vi "setUp.vi"(8 "error in (no error)":errorcluster, 11 "reference in":refnum<class "Engine Simulation IO System Tests.lvclass">) -> (0 "error out":errorcluster, 3 "reference out":refnum<class "Engine Simulation IO System Tests.lvclass">)   [LabVIEW 2015, in "Engine Simulation IO System Tests.lvclass"]
doc: "setUp runs prior to the test method during test execution. Use this method to initialize any object data required by your tests."
uses:
  Engine Simulation IO System Tests.lvclass
  NationalInstruments.VeriStand.SystemDefinitionAPI
  Engine Simulation IO System Tests.lvclass/Engine Simulation IO System Tests.ctl
  <userlib>/_OpenG.lib/file/file.llb/Append Path to Root if Relative - Scalar__ogtk.vi
  <vilib>/addons/_JKI Toolkits/VI Tester/TestCase.llb/TestCase.lvclass
  Scripting API/Engine Simulation Toolkit Scripting API.lvlib
  System Explorer/Engine Simulation Toolkit System Explorer.lvlib
  niveristand-custom-device-testing-tools/VeriStandTestUtilities/VeriStandTestUtilities.lvlib
panel:
  in  "System Definition File":path=path "Assets/estksysdef.nivssdf"
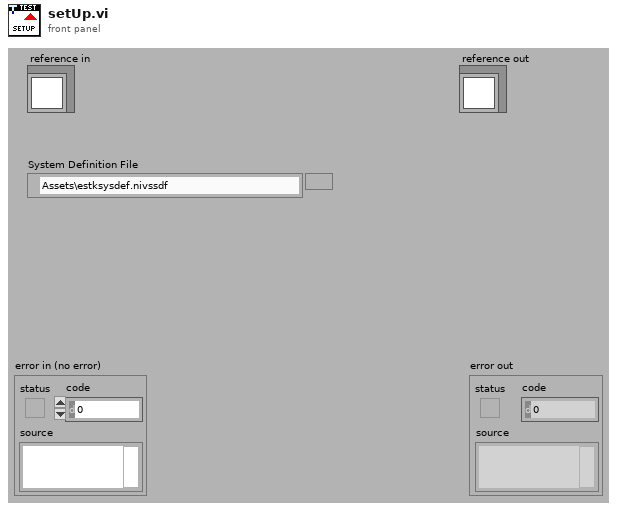
[diagram p1: front panel]
types:
  T1 = typedef "VeriStandTestUtilities.lvlib/SystemDefinitionInformation.ctl" = cluster{"Path":path, "Target Information List":T2[]}
  T2 = typedef "VeriStandTestUtilities.lvlib/TargetInformation.ctl" = cluster{"Name":string, "IP Address":string, "Operating System":string, "Target Rate":dbl, "Chassis List":T3[], "Custom Device List":string[]}
  T3 = typedef "VeriStandTestUtilities.lvlib/ChassisInformation.ctl" = cluster{"Name":string, "Devices":string[]}
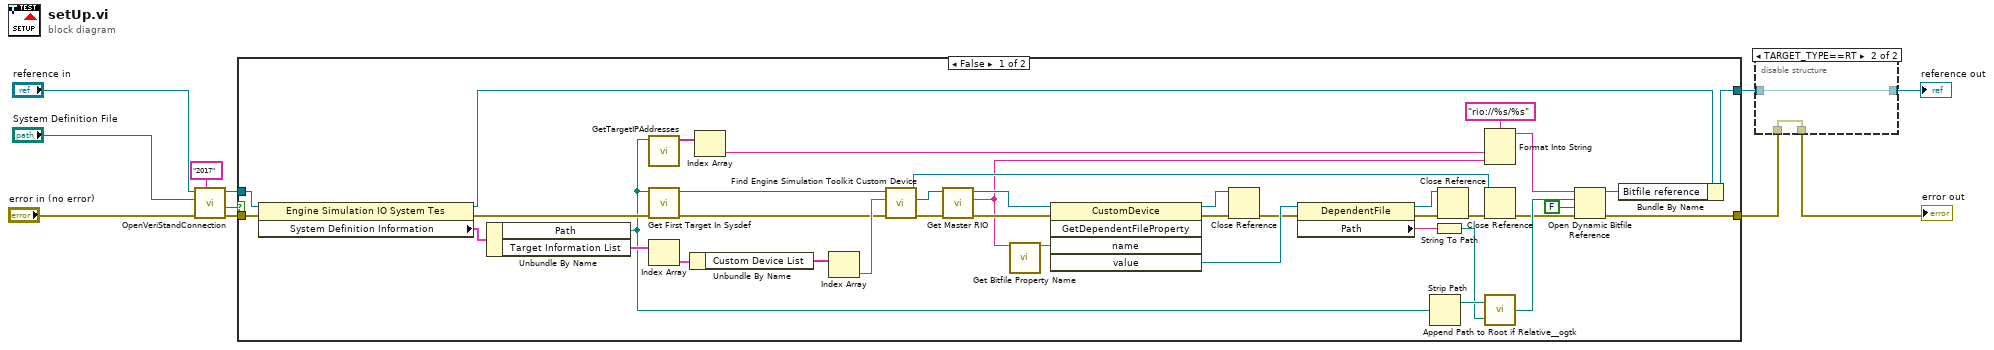
[diagram p0: block diagram]
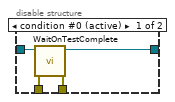
[diagram p3: hidden frame]
diagram:
  n1 = call-dynamic "OpenVeriStandConnection.vi"("Minimum VeriStand Version (2015)"="2017", "error in (no error)"="error in (no error)", "System Definition File"="System Definition File", "VeriStand Test Case in"="reference in") -> ("error out"=w5:errorcluster, "Open Skipped"=w1:bool, "VeriStand Test Case out"=w6:refnum<class "Engine Simulation IO System Tests.lvclass">)  [unwired: 5 in]
  n2 = case shown="False" w1 {
    tunnel: [w50 w51] -> w9
    tunnel: w6 -> [w49 w51]
    tunnel: w5 -> [w48 w52]
    tunnel: [w20 w52] -> w4
    frame False {
      n3 = property class="Engine Simulation IO System Tes"(reference=w49, error in=w48) -> (reference out=w12:refnum<class "Engine Simulation IO System Tests.lvclass">, error out=w46:errorcluster, "System Definition Information"=w47:T1)
      n4 = Unbundle By Name(w47) -> ("Path"=w16:path, "Target Information List"=w26:T2[])
      n5 = call "GetTargetIPAddresses.vi"("absolute system definition file"=w16) -> ("ip addresses"=w15:string[])  [unwired: 9 in, 1 out]
      n6 = call "Get First Target In Sysdef.vi"("error in (no error)"=w46, "Sysdef Path"=w16) -> ("error out"=w24:errorcluster, "Target"=w25:refnum<k24>)  [unwired: 8 in]
      n7 = Index Array(array=w26) -> (element=w45:T2)  [unwired: 1 in]
      n8 = Unbundle By Name(w45) -> ("Custom Device List"=w44:string[])
      n9 = Index Array(array=w15) -> (element=w14:string)  [unwired: 1 in]
      n10 = Index Array(array=w44) -> (element=w43:string)  [unwired: 1 in]
      n11 = call "Find Engine Simulation Toolkit Custom Device.vi"("error in (no error)"=w24, "Name"=w43, "Target in"=w25) -> ("error out"=w38:errorcluster, "EST Custom Device"=w40:refnum<k24>, "Target out"=w42:refnum<k24>)  [unwired: 6 in]
      n12 = call "Get Master RIO.vi"("error in (no error)"=w38, "EST Custom Device in"=w40) -> ("error out"=w37:errorcluster, "RIO Device Address"=w17:string, "EST Custom Device out"=w35:refnum<k24>)  [unwired: 7 in]
      n13 = call "Get Bitfile Property Name.vi"("RIO Device Address in"=w17) -> ("Bitfile Property Name"=w39:string)  [unwired: 10 in]
      n14 = invoke class="CustomDevice" method="GetDependentFileProperty"(reference=w35, error in=w37, "name"=w39) -> (reference out=w33:refnum<k24>, error out=w34:errorcluster, "value"=w41:refnum<k24>)  [unwired: 2 in, 2 out]
      n15 = Close Reference(reference=w33, error in (no error)=w34) -> (error out=w32:errorcluster)
      n16 = property class="DependentFile"(reference=w41, error in=w32) -> (reference out=w30:refnum<k24>, error out=w31:errorcluster, "Path"=w36:string)
      n17 = Strip Path(path=w16) -> (stripped path=w28:path)  [unwired: 1 out]
      n18 = String To Path(string=w36) -> (path=w27:path)
      n19 = Close Reference(reference=w30, error in (no error)=w31) -> (error out=w29:errorcluster)
      n20 = Format Into String(format string="rio://%s/%s", w14, w17) -> (resulting string=w13:string)  [unwired: 2 in, 1 out]
      n21 = Close Reference(reference=w42, error in (no error)=w29) -> (error out=w19:errorcluster)
      n22 = call-poly <userlib>:"Append Path to Root if Relative__ogtk.vi"("Absolute or Relative Path"=w27, "Root Path"=w28) -> ("Absolute or Appended Path"=w22:path)
      n23 = Open Dynamic Bitfile Reference(0:w13, 1:w22, 2:FALSE ("Run When Loaded"), 3:w19) -> (5:w21:refnum<k20>, 8:w20:errorcluster)  [unwired: 1 in]
      n24 = Bundle By Name(cluster=w12, "Bitfile reference"=w21) -> (w50:refnum<class "Engine Simulation IO System Tests.lvclass">)
    }
    frame True {
    }
  }
  n25 = disable-structure shown="TARGET_TYPE==RT" {
    disable-tunnel: w4 -> [w56 w57]
    disable-tunnel: [w55 w57] -> w11
    disable-tunnel: [w54 w58] -> w10
    disable-tunnel: w9 -> [w53 w58]
    frame condition #0 (active) {
      n26 = call <vilib>:"WaitOnTestComplete.vi"("error in (no error)"=w56, "TestCase in"=w53) -> ("error out"=w55:errorcluster, "TestCase out"=w54:refnum<class "Engine Simulation IO System Tests.lvclass">)  [unwired: 8 in]
    }
    frame condition #1 {
    }
  }
  "error out" <- w11
  "reference out" <- w10
